vi "Filter Group Names by Type.vi"(11 "Channel Group Details":cluster{"Group Name":string, "Type":string}[](array[cluster])) -> (1 "Output Groups":string[](array[string]), 3 "Input Groups":string[](array[string]))   [LabVIEW 2026]
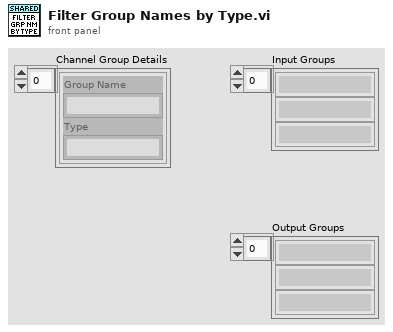
[diagram p1: front panel]
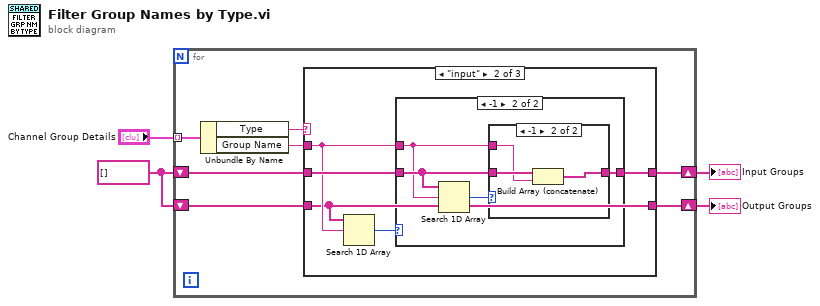
[diagram p0: block diagram]
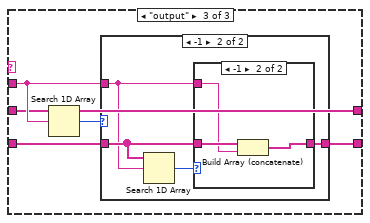
[diagram p5: hidden frame]
diagram:
  w3 = string[] []
  n1 = for {
    tunnel: "Channel Group Details" -> [w11] mode=indexing
    shift-right: [w6] -> w2
    shift-left: w3 -> [w8]
    shift-right: [w5] -> w1
    shift-left: w3 -> [w7]
    n2 = Unbundle By Name(w11) -> ("Type"=w10:string, "Group Name"=w9:string)
    n3 = case shown="\"input\"" w10 {
      tunnel: w9 -> [_ w16 w31]
      tunnel: w8 -> [w13 w17 w28]
      tunnel: w7 -> [w12 w14 w30]
      tunnel: [w13 w15 w28] -> w6
      tunnel: [w12 w14 w29] -> w5
      frame Default {
      }
      frame "input" {
        n4 = Search 1D Array(1D array=w14, element=w16) -> (index of element=w18:i32)  [unwired: 1 in]
        n5 = case shown="-1" w18 {
          tunnel: w17 -> [w19 w22]
          tunnel: w16 -> [_ w20]
          tunnel: [w19 w21] -> w15
          frame 0, Default {
          }
          frame -1 {
            n6 = Search 1D Array(1D array=w22, element=w20) -> (index of element=w23:i32)  [unwired: 1 in]
            n7 = case shown="-1" w23 {
              tunnel: w22 -> [w24 w27]
              tunnel: w20 -> [_ w26]
              tunnel: [w24 w25] -> w21
              frame 0, Default {
              }
              frame -1 {
                n8 = Build Array (concatenate)(w27, w26) -> (w25:string[])
              }
            }
          }
        }
      }
      frame "output" {
        n9 = Search 1D Array(1D array=w28, element=w31) -> (index of element=w32:i32)  [unwired: 1 in]
        n10 = case shown="-1" w32 {
          tunnel: w30 -> [w33 w36]
          tunnel: w31 -> [_ w34]
          tunnel: [w33 w35] -> w29
          frame 0, Default {
          }
          frame -1 {
            n11 = Search 1D Array(1D array=w36, element=w34) -> (index of element=w37:i32)  [unwired: 1 in]
            n12 = case shown="-1" w37 {
              tunnel: w36 -> [w38 w41]
              tunnel: w34 -> [_ w40]
              tunnel: [w38 w39] -> w35
              frame 0, Default {
              }
              frame -1 {
                n13 = Build Array (concatenate)(w41, w40) -> (w39:string[])
              }
            }
          }
        }
      }
    }
  }
  "Input Groups" <- w2
  "Output Groups" <- w1
